vi "Text Prompt.vi"(6 "Password? (F)":bool, 8 "error in (no error)":errorcluster, 9 "Default":string, 10 "Prompt":string, 11 "UI in":refnum<class "UI.lvclass">) -> (0 "error out":errorcluster, 2 "Response":string, 3 "UI out":refnum<class "UI.lvclass">)   [LabVIEW 2020, in "neg-pkg.lvlib" / "UI.lvclass"]
uses:
  UI.lvclass
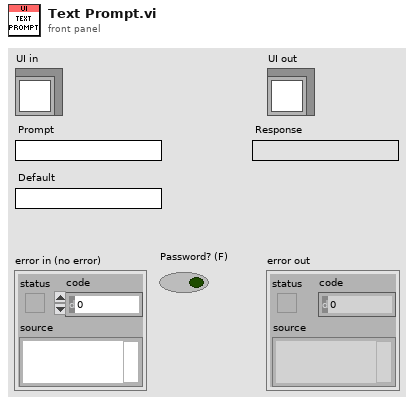
[diagram p1: front panel]
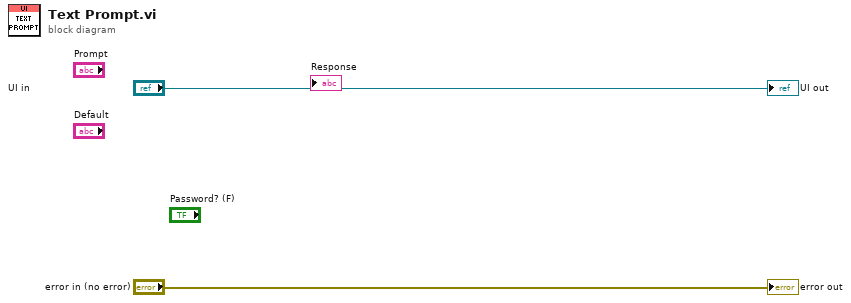
[diagram p0: block diagram]
diagram:
  "error out" <- "error in (no error)"
  "UI out" <- "UI in"
